vi "Board_Global_Var.vi"() -> ()   [LabVIEW 2019]
panel:
  in  "Save Results":bool
  out "ResDir":path
  in  "Status Read En":bool
  out "Pulser error":errorcluster
  in  "Pulser VISA":refnum<visa-resource-name>
  in  "Session Log ref":refnum<vi>
  in  "Error Messages":string[](array[string])=["INVALID START OF FRAME", "INVALID HEADER", "INVALID WRITE END", "INVALID STATE"]
  in  "Status Messages":string[](array[string])=["CONTROLLER IDLE", "WAITING HEADER", "WAITING NB OF RD WORDS", "WAITING NB OF WR WORDS", "WAITING WR DATA", "RECEIVED CONTROL CMD", "READ IN PROGRESS", "WRITE IN PROGRESS", "READ COMPLETED", "WRITE COMPLETED", "STATUS READ INITIATED", "STATUS READ COMPLETED"]
  out "Board error":errorcluster
  in  "Board VISA":refnum<visa-resource-name>
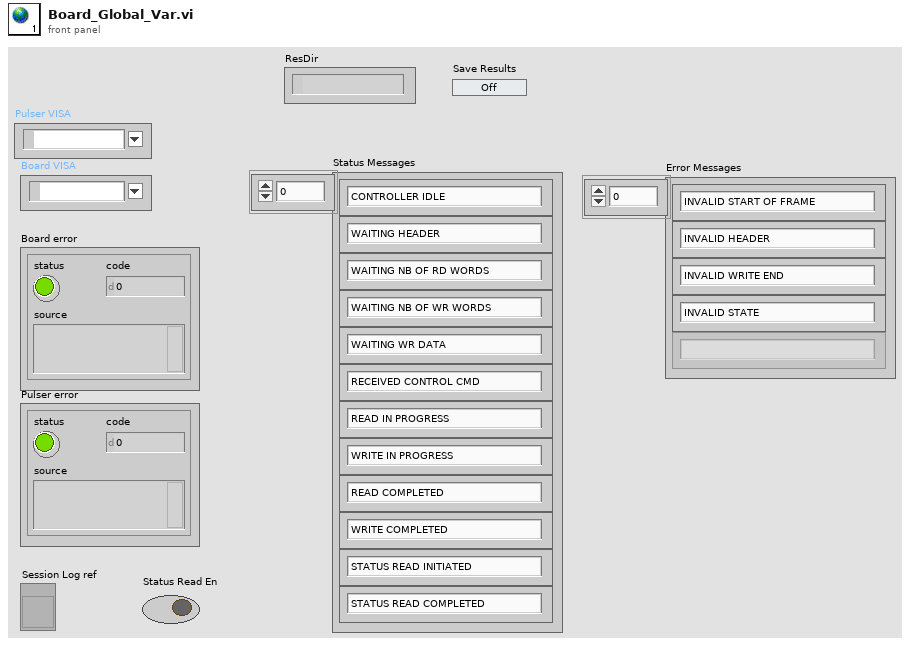
[diagram p1: front panel]
diagram:
